vi "GetStatusLine.vi"(3 "Status":T1[](array[typedef])) -> (0 "all good?":bool, 1 "Status":string)   [LabVIEW 2016]
doc: "Gets the status of the master"
uses:
  MyState.ctl
  _ROSDefinition.vi
panel:
  out "h(x)":i32[](array[numeric])
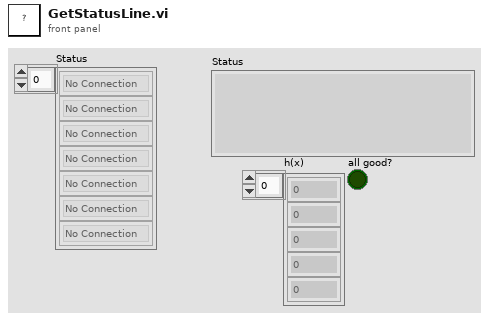
[diagram p1: front panel]
types:
  T1 = typedef "MyState.ctl" = enum16{"No Connection", "Registered", "Connected", "Close"}
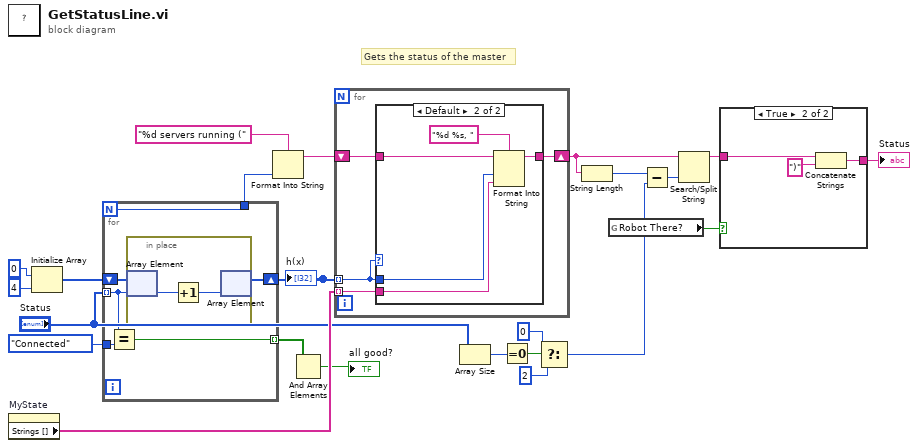
[diagram p0: block diagram]
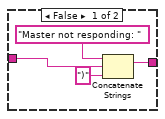
[diagram p2: hidden frame]
diagram:
  # "Gets the status of the master"
  n1 = property on="MyState" class="Enum (strict)"() -> ("Strings []"=w23:string[])  [unwired: 2 in, 2 out]
  n2 = Initialize Array(u8 0 ("element"), 4 ("dimension size")) -> (w19:u8[])
  n3 = for {
    N -> [w27]
    shift-right: [w28] -> w7
    shift-left: w19 -> [w29]
    tunnel: "Status" -> [w25] mode=indexing
    tunnel: [w27] -> w12
    tunnel: MyState."Connected" ("MyState") -> [w26]
    tunnel: [w24] -> w9 mode=indexing
    n4 = Equal?(x=w25, y=w26) -> (x = y?=w24:bool)
    n5 = in-place {
      n6 = in-place-array #1(w29, w25) -> (w31:u8)
      n7 = Increment(x=w31) -> (x+1=w30:u8)
      n8 = in-place-array #1(w30) -> (w28:u8[])  [unwired: 1 out]
    }
  }
  "h(x)" <- w7
  n9 = Format Into String(format string="%d servers running (" ("regular expression"), w12) -> (resulting string=w20:string)  [unwired: 2 in, 1 out]
  n10 = And Array Elements(Boolean array=w9) -> (logical AND=→"all good?":bool)
  n11 = for {
    shift-right: [w34] -> w15
    shift-left: w20 -> [w35]
    tunnel: w23 -> [w33] mode=indexing
    tunnel: w7 -> [w32] mode=indexing
    n12 = case shown="Default" w32 {
      tunnel: w35 -> [w36 w41]
      tunnel: [w36 w40] -> w34
      tunnel: w33 -> [_ w38]
      tunnel: w32 -> [_ w37]
      frame 0 {
      }
      frame Default {
        n13 = Format Into String(format string="%d %s, ", initial string=w41, w37, w38) -> (resulting string=w40:string)  [unwired: 1 in, 1 out]
      }
    }
  }
  n14 = Array Size(array="Status") -> (size(s)=w6:i32)
  n15 = Equal To 0?(x=w6) -> (x = 0?=w5:bool)
  n16 = Select(t=0 ("y"), s=w5, f=2 ("y")) -> (s? t:f=w2:i32)
  n17 = String Length(string=w15) -> (length=w14:i32)
  n18 = global read "_ROSDefinition.vi" "Robot There?"() -> (w11:bool)
  n19 = Subtract(x=w14, y=w2) -> (x-y=w13:i32)
  n20 = Search/Split String(string=w15, offset (0)=w13) -> (substring before match=w16:string)  [unwired: 1 in, 2 out]
  n21 = case shown="True" w11 {
    tunnel: [w43 w47] -> w22
    tunnel: w16 -> [w44 w46]
    frame False {
      n22 = Concatenate Strings("Master not responding: ", w44, ")" ("string")) -> (w43:string)
    }
    frame True {
      n23 = Concatenate Strings(w46, ")" ("string")) -> (w47:string)
    }
  }
  "Status" <- w22
